vi "SimpleVoltageBiasPoin.vi"(0 "VBias1":dbl, 1 "VBias2":dbl, 2 "VBias3":dbl, 3 "CC1":dbl, 4 "CC2":dbl, 5 "CC3":dbl, 6 "CR1":dbl, 7 "CR2":dbl, 9 "CR3":dbl, 14 "VISA resource name":refnum<visa-resource-name>, 16 "error in (no error)":errorcluster) -> (15 "VISA resource name out":refnum<visa-resource-name>, 17 "error out":errorcluster, 20 "T1":string, 21 "T2":string, 22 "T3":string, 23 "Current, bundled":string)   [LabVIEW 2021]
panel:
  out "Pushed_string":string
  # "Data on the equipment is pushed to an output buffer, this buffer can be read from, in order (I currently beliveve)"
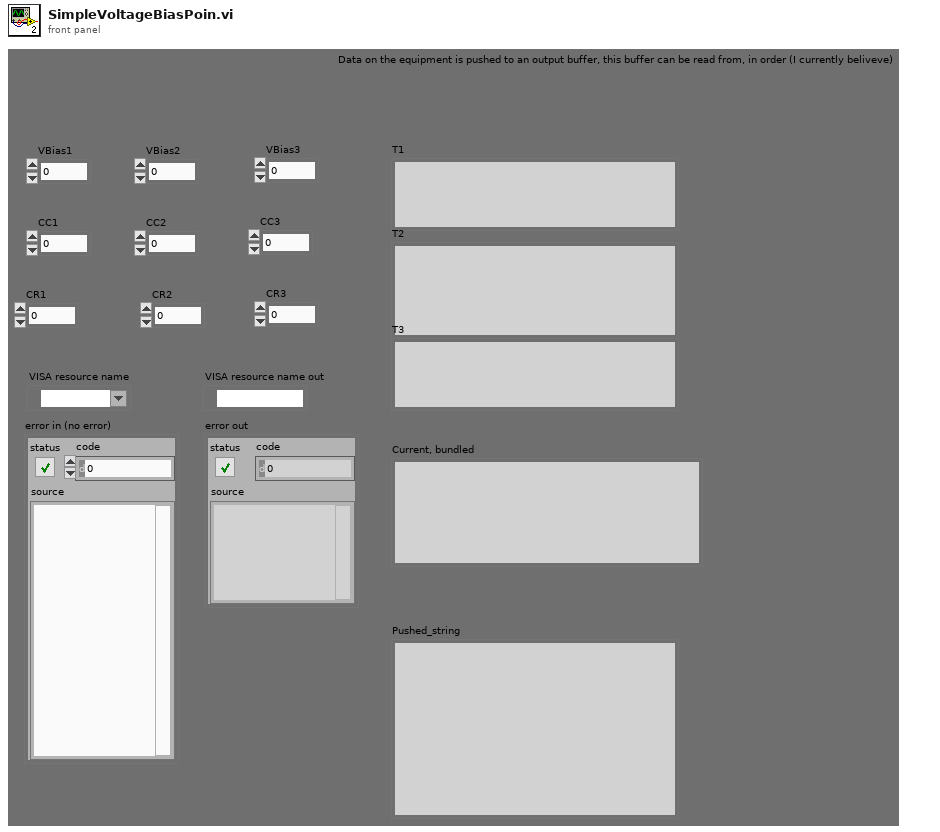
[diagram p1: front panel]
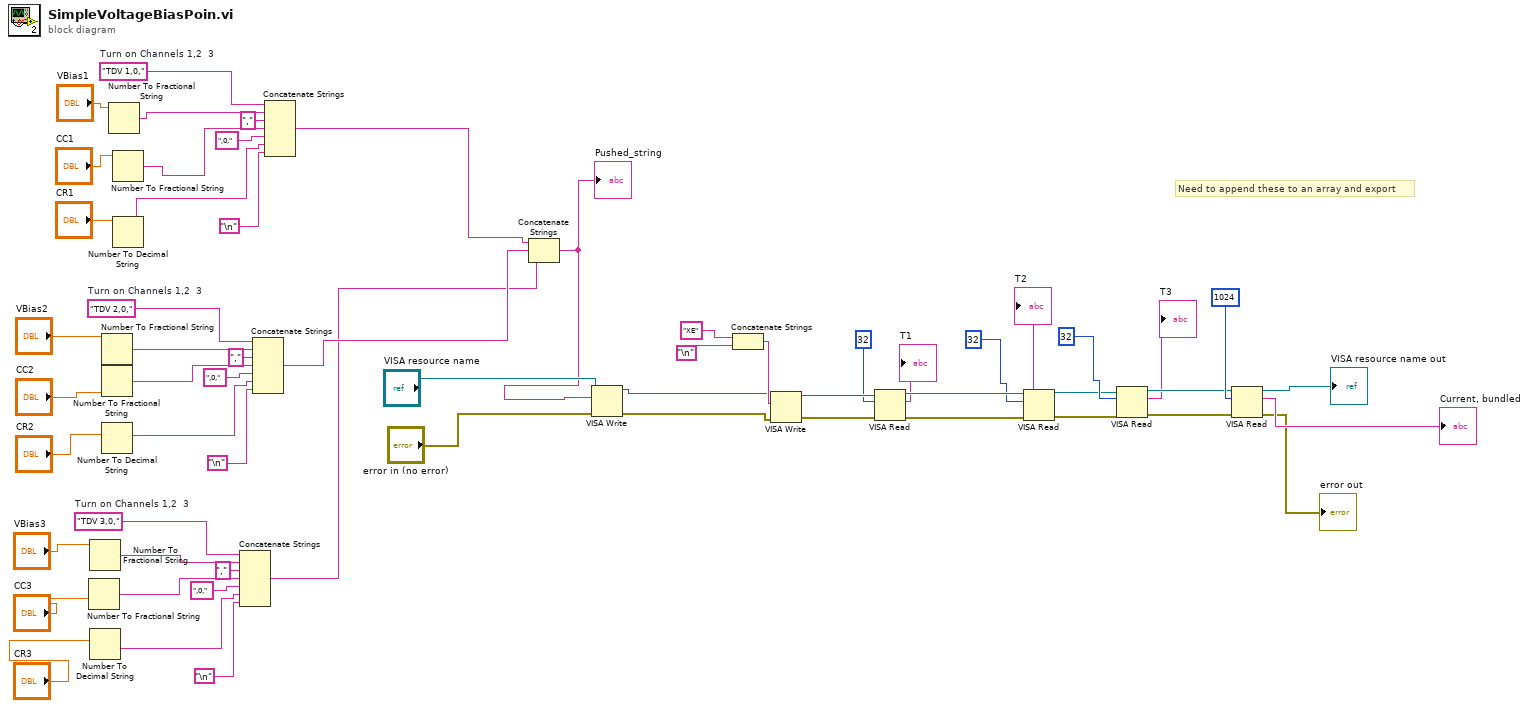
[diagram p0: block diagram]
diagram:
  w41 = "TDV 3,0,"  # Turn on Channels 1,2  3
  w51 = "TDV 2,0,"  # Turn on Channels 1,2  3
  w59 = "TDV 1,0,"  # Turn on Channels 1,2  3
  # "Need to append these to an array and export"
  n1 = Number To Fractional String(number="CC3") -> (F-format string=w38:string)  [unwired: 3 in]
  n2 = Number To Fractional String(number="VBias3") -> (F-format string=w40:string)  [unwired: 3 in]
  n3 = Number To Decimal String(number="CR3") -> (decimal integer string=w36:string)  [unwired: 1 in]
  n4 = Number To Fractional String(number="VBias2") -> (F-format string=w50:string)  [unwired: 3 in]
  n5 = Number To Fractional String(number="CC2") -> (F-format string=w48:string)  [unwired: 3 in]
  n6 = Number To Decimal String(number="CR2") -> (decimal integer string=w46:string)  [unwired: 1 in]
  n7 = Number To Fractional String(number="VBias1") -> (F-format string=w2:string)  [unwired: 3 in]
  n8 = Number To Fractional String(number="CC1") -> (F-format string=w3:string)  [unwired: 3 in]
  n9 = Number To Decimal String(number="CR1") -> (decimal integer string=w53:string)  [unwired: 1 in]
  n10 = Concatenate Strings(w41, w40, "," ("string"), w38, ",0," ("string"), w36, "\n") -> (w8:string)
  n11 = Concatenate Strings(w51, w50, "," ("string"), w48, ",0," ("string"), w46, "\n") -> (w9:string)
  n12 = Concatenate Strings(w59, w2, "," ("string"), w3, ",0," ("string"), w53, "\n") -> (w10:string)
  n13 = Concatenate Strings(w10, w9, w8) -> (w5:string)
  "Pushed_string" <- w5
  n14 = VISA Write(VISA resource name="VISA resource name", write buffer=w5, error in (no error)="error in (no error)") -> (VISA resource name out=w7:refnum<visa-resource-name>, error out=w6:errorcluster)  [unwired: 1 out]
  n15 = Concatenate Strings("XE" ("string"), "\n") -> (w31:string)
  n16 = VISA Write(VISA resource name=w7, write buffer=w31, error in (no error)=w6) -> (VISA resource name out=w28:refnum<visa-resource-name>, error out=w27:errorcluster)  [unwired: 1 out]
  n17 = VISA Read(VISA resource name=w28, byte count=u32 32, error in (no error)=w27) -> (VISA resource name out=w25:refnum<visa-resource-name>, read buffer=→"T1":string, error out=w24:errorcluster)  [unwired: 1 out]
  n18 = VISA Read(VISA resource name=w25, byte count=u32 32, error in (no error)=w24) -> (VISA resource name out=w21:refnum<visa-resource-name>, read buffer=→"T2":string, error out=w20:errorcluster)  [unwired: 1 out]
  n19 = VISA Read(VISA resource name=w21, byte count=u32 32, error in (no error)=w20) -> (VISA resource name out=w18:refnum<visa-resource-name>, read buffer=→"T3":string, error out=w13:errorcluster)  [unwired: 1 out]
  n20 = VISA Read(VISA resource name=w18, byte count=u32 1024, error in (no error)=w13) -> (VISA resource name out=→"VISA resource name out":refnum<visa-resource-name>, read buffer=→"Current, bundled":string, error out=→"error out":errorcluster)  [unwired: 1 out]
